vi "Check Channel and Enable.vi"(8 "error in (no error)":errorcluster, 11 "Scan Data Process in":T1) -> (0 "error out":errorcluster, 3 "Scan Data Process out":T1)   [LabVIEW 2015, in "Exposure Process.lvlib"]
uses:
  Exposure Process.lvlib
  Control_Scan Data Process.ctl
  <vilib>/addons/PointValueMap/controls/PointMap.ctl
  Control_EXP Information.ctl
  Control_File Save Setup.ctl
  Control_Enable and Path.ctl
  Control_ICM Export Setting.ctl
  ConfigHelper/ConfigHelper.lvlib
  <vilib>/addons/PointValueMap/PointValueMap.lvlib
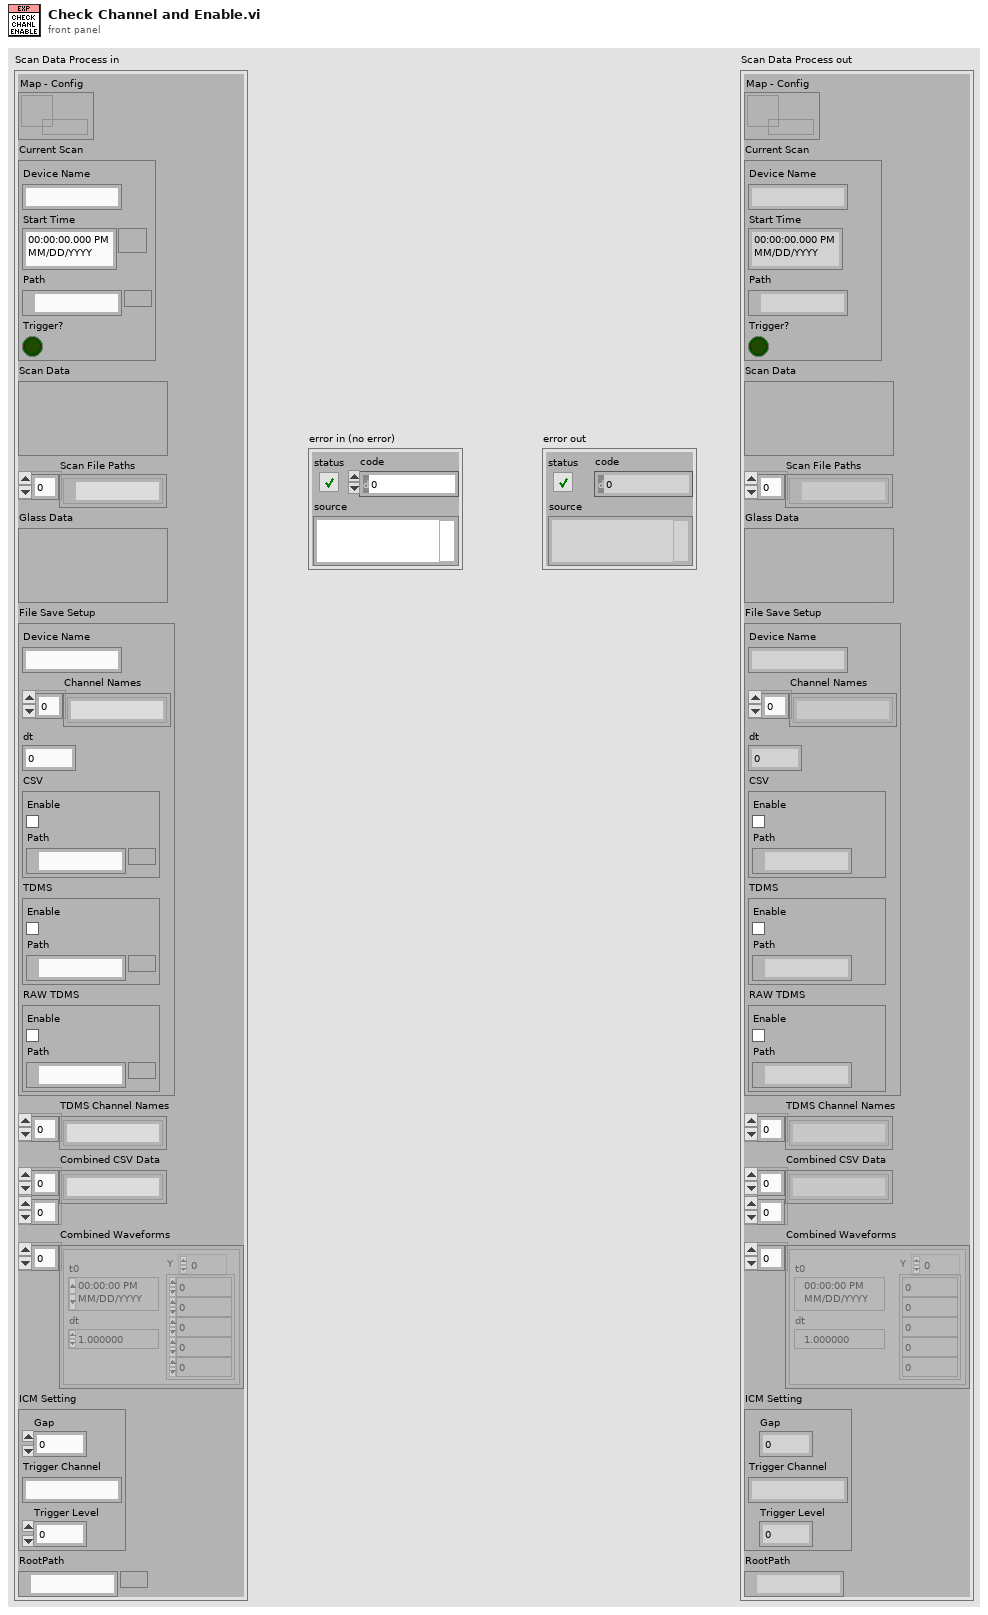
[diagram p1: front panel]
types:
  T1 = typedef "Exposure Process.lvlib/Control_Scan Data Process.ctl" = cluster{"Map - Config":T2, "Current Scan":T3, "Scan Data":variant, "Scan File Paths":path[], "Glass Data":variant, "File Save Setup":T4, "TDMS Channel Names":string[], "Combined CSV Data":string[][], "Combined Waveforms":waveform(dbl)[], "ICM Setting":T6, "RootPath":path}
  T2 = typedef "PointValueMap.lvlib/PointMap.ctl" = refnum<data-value>
  T3 = typedef "Exposure Process.lvlib/Control_EXP Information.ctl" = cluster{"Device Name":string, "Start Time":timestamp, "Path":path, "Trigger?":bool}
  T4 = typedef "Exposure Process.lvlib/Control_File Save Setup.ctl" = cluster{"Device Name":string, "Channel Names":string[], "dt":dbl, "CSV":T5, "TDMS":T5, "RAW TDMS":T5}
  T5 = typedef "Exposure Process.lvlib/Control_Enable and Path.ctl" = cluster{"Enable":bool, "Path":path}
  T6 = typedef "Exposure Process.lvlib/Control_ICM Export Setting.ctl" = cluster{"Gap":dbl, "Trigger Channel":string, "Trigger Level":dbl}
  T7 = typedef "ConfigHelper.lvlib/Control_Export Setup.ctl" = cluster{"Device Name":string, "Export CSV":bool, "Export TDMS":bool, "Export RAW TDMS":bool, "Channel Names":string[]}
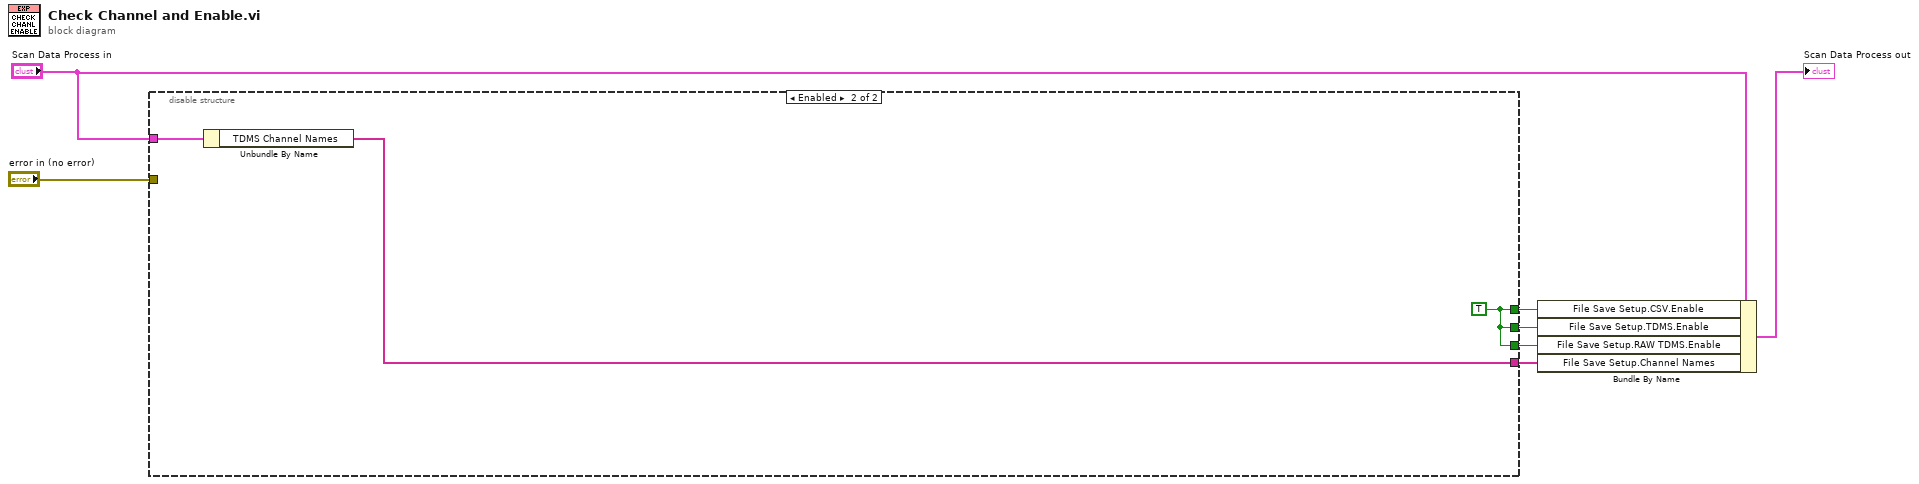
[diagram p0: block diagram]
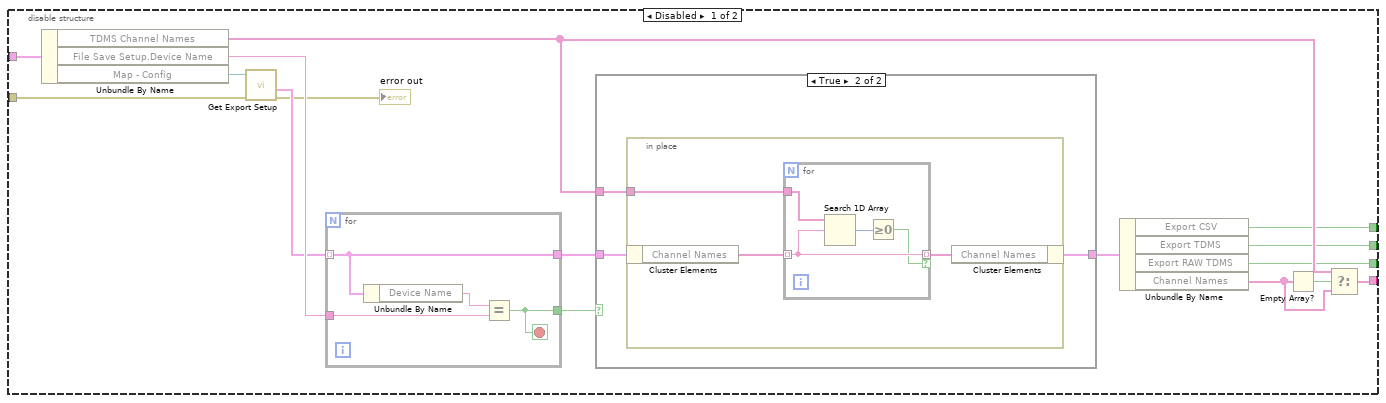
[diagram p2: hidden frame]
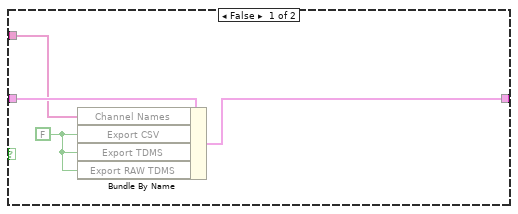
[diagram p3: hidden frame]
diagram:
  n1 = disable-structure shown="Enabled" {
    disable-tunnel: [w14 w44] -> w7
    disable-tunnel: [w13 w44] -> w6
    disable-tunnel: [w12 w44] -> w5
    disable-tunnel: [w11 w42] -> w4
    disable-tunnel: "error in (no error)" -> [w10 _]
    disable-tunnel: "Scan Data Process in" -> [w8 w43]
    frame Disabled {
      n2 = Unbundle By Name(w8) -> ("TDMS Channel Names"=w17:string[], "File Save Setup.Device Name"=w21:string, "Map - Config"=w19:T2)
      n3 = call "Get Export Setup.vi"("error in (no error)"=w10, "Map"=w19) -> ("error out"=→"error out":errorcluster, "Export Setup"=w20:T7[])  [unwired: 7 in, 1 out]
      n4 = for {
        tunnel: w20 -> [w39] mode=indexing
        tunnel: w21 -> [w41]
        tunnel: [w39] -> w22
        tunnel: [w38] -> w23
        stop <- w38 stop-if-true
        n5 = Unbundle By Name(w39) -> ("Device Name"=w40:string)
        n6 = Equal?(x=w40, y=w41) -> (x = y?=w38:bool)
      }
      n7 = case shown="True" w23 {
        tunnel: w22 -> [w27 w30]
        tunnel: w17 -> [w26 w29]
        tunnel: [w25 w28] -> w15
        frame False {
          w24 = FALSE ("Export CSV")
          n8 = Bundle By Name(cluster=w27, "Channel Names"=w26, "Export CSV"=w24, "Export TDMS"=w24, "Export RAW TDMS"=w24) -> (w25:T7)
        }
        frame True {
          n9 = in-place {
            in-place-border: w29 -> [w32]
            n10 = in-place-cluster #1(w30) -> ("Channel Names"=w33:string[])
            n11 = for {
              tunnel: w33 -> [w36] mode=indexing
              tunnel: [w36] -> w31 mode=indexing if=w35
              tunnel: w32 -> [w34]
              n12 = Search 1D Array(1D array=w34, element=w36) -> (index of element=w37:i32)  [unwired: 1 in]
              n13 = Greater Or Equal To 0?(x=w37) -> (x >= 0?=w35:bool)
            }
            n14 = in-place-cluster #1("Channel Names"=w31) -> (w28:T7)
          }
        }
      }
      n15 = Unbundle By Name(w15) -> ("Export CSV"=w14:bool, "Export TDMS"=w13:bool, "Export RAW TDMS"=w12:bool, "Channel Names"=w16:string[])
      n16 = Empty Array?(array=w16) -> (empty?=w18:bool)
      n17 = Select(t=w17, s=w18, f=w16) -> (s? t:f=w11:string[])
    }
    frame Enabled {
      w44 = TRUE ("Export CSV")
      n18 = Unbundle By Name(w43) -> ("TDMS Channel Names"=w42:string[])
    }
  }
  n19 = Bundle By Name(cluster="Scan Data Process in", "File Save Setup.CSV.Enable"=w7, "File Save Setup.TDMS.Enable"=w6, "File Save Setup.RAW TDMS.Enable"=w5, "File Save Setup.Channel Names"=w4) -> (→"Scan Data Process out":T1)
